vi "Scratch.vi"() -> ()   [LabVIEW 2020, in "VolatusGUIElements.lvlib" / "2WayValveV.lvclass"]
uses:
  2WayValveV.lvclass
  2WayValveV.lvclass/2WayValveV.ctl
  VolatusGUIControls/2WayValveH.ctl
  VolatusGUIControls/VolatusGUIControls.lvlib
  Picture.ctl
  Command Pictures.ctl
  Feedback Pictures.ctl
  Energized Pictures.ctl
  Valve Pictures.ctl
  Values.ctl
  Channel State.ctl
  Unused Element.ctl
panel:
  in  "Unused":T1
  in  "Valve Pictures":T2={"Command"={"Error"=enum."InError", "Config"=enum."InConfig", "Stale"=enum."InStale", "Close"=enum."InClose", "Open"=enum."InOpen", "TranClose"=enum."Blank", "TranOpen"=enum."Blank"}, "Feedback"={"Error"=enum."OutError", "Config"=enum."OutConfig", "Stale"=enum."OutStale", "Closed"=enum."OutClose", "Open"=enum."OutOpen", "TranClose"=enum."OutTranClose", "TranOpen"=enum."Blank"}, "Energized"={"Error"=enum."EnError", "Config"=enum."EnConfig", "Stale"=enum."EnStale", "False"=enum."EnOff", "True"=enum."EnOn"}}
  in  "Values":T7={"Command"={"Value"=FALSE, "Stale"=FALSE, "Config"=FALSE, "Error"=FALSE, "Prev"=FALSE}, "CmdFB"={"Value"=FALSE, "Stale"=FALSE, "Config"=FALSE, "Error"=FALSE, "Prev"=FALSE}, "Closed"={"Value"=TRUE, "Stale"=FALSE, "Config"=FALSE, "Error"=FALSE, "Prev"=FALSE}, "Open"={"Value"=FALSE, "Stale"=FALSE, "Config"=FALSE, "Error"=FALSE, "Prev"=FALSE}, "Energized"={"Value"=FALSE, "Stale"=FALSE, "Config"=FALSE, "Error"=FALSE, "Prev"=FALSE}}
  in  "2WayValve":T9={"Picture"=bytes[12402], "Command"=FALSE}
  # "Abort to stop"
  # "Config options below"
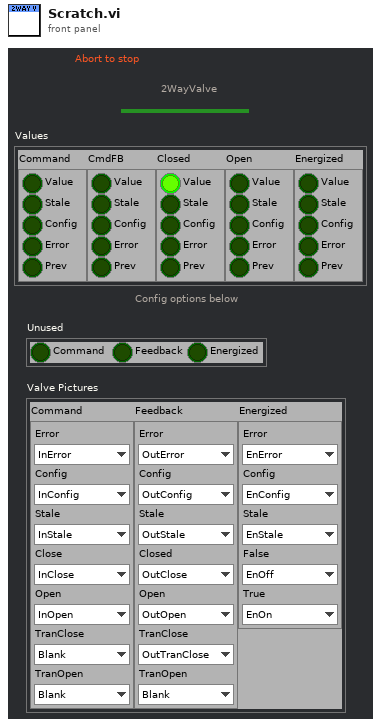
[diagram p1: front panel]
types:
  T1 = typedef "VolatusGUIElements.lvlib/2WayValveV.lvclass/Unused Element.ctl" = cluster{"Command":bool, "Feedback":bool, "Energized":bool}
  T2 = typedef "VolatusGUIElements.lvlib/2WayValveV.lvclass/Valve Pictures.ctl" = cluster{"Command":T3, "Feedback":T5, "Energized":T6}
  T3 = typedef "VolatusGUIElements.lvlib/2WayValveV.lvclass/Command Pictures.ctl" = cluster{"Error":T4, "Config":T4, "Stale":T4, "Close":T4, "Open":T4, "TranClose":T4, "TranOpen":T4}
  T4 = typedef "VolatusGUIElements.lvlib/2WayValveV.lvclass/Picture.ctl" = enum16{"Blank", "OutClose", "OutOpen", "OutTranClose", "OutTranOpen", "OutConfig", "OutStale", "OutError", "InClose", "InOpen", "InTranClose", "InTranOpen", "InConfig", "InStale", "InError", "EnOff", "EnOn", "EnConfig", "EnStale", "EnError"}
  T5 = typedef "VolatusGUIElements.lvlib/2WayValveV.lvclass/Feedback Pictures.ctl" = cluster{"Error":T4, "Config":T4, "Stale":T4, "Closed":T4, "Open":T4, "TranClose":T4, "TranOpen":T4}
  T6 = typedef "VolatusGUIElements.lvlib/2WayValveV.lvclass/Energized Pictures.ctl" = cluster{"Error":T4, "Config":T4, "Stale":T4, "False":T4, "True":T4}
  T7 = typedef "VolatusGUIElements.lvlib/2WayValveV.lvclass/Values.ctl" = cluster{"Command":T8, "CmdFB":T8, "Closed":T8, "Open":T8, "Energized":T8}
  T8 = typedef "VolatusGUIElements.lvlib/2WayValveV.lvclass/Channel State.ctl" = cluster{"Value":bool, "Stale":bool, "Config":bool, "Error":bool, "Prev":bool}
  T9 = typedef "VolatusGUIControls.lvlib/2WayValveH.ctl" = cluster{"Picture":picture, "Command":bool}
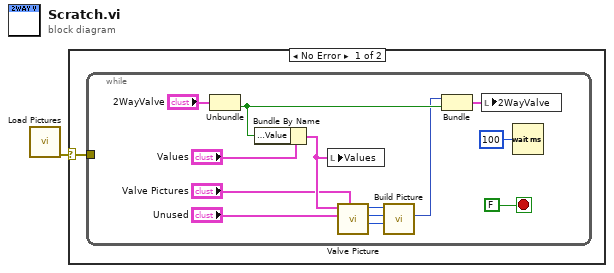
[diagram p0: block diagram]
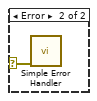
[diagram p2: hidden frame]
diagram:
  n1 = call "Load Pictures.vi"() -> ("error out"=w1:errorcluster)  [unwired: 11 in]
  n2 = case shown="No Error" w1 {
    selector: w1 -> [w2 w16]
    frame No Error {
      n3 = while {
        tunnel: w2 -> [_]
        stop <- FALSE stop-if-true
        n4 = Unbundle("2WayValve") -> ("Command"=w11:bool)  [unwired: 1 out]
        n5 = Bundle By Name(cluster="Values", "Command.Value"=w11) -> (w9:T7)
        n6 = local write "Values"(w9) -> ()
        n7 = call "Valve Picture.vi"("Valve Pictures"="Valve Pictures", "Unused Element"="Unused", "Values"=w9) -> ("Energized Picture"=w4:T4, "Feedback Picture"=w5:T4, "Command Picture"=w6:T4)  [unwired: 6 in]
        n8 = call "Build Picture.vi"("Energized Picture"=w4, "Feedback Picture"=w5, "Command Picture"=w6) -> ("Valve Picture"=w3:picture)  [unwired: 8 in]
        n9 = Bundle("Valve Picture"=w3, "Command"=w11) -> (w10:cluster{"Valve Picture":picture, "Command":bool})  [unwired: 1 in]
        n10 = local write "2WayValve"(w10) -> ()
        n11 = Wait (ms)(milliseconds to wait=u32 100) -> ()  [unwired: 1 out]
      }
    }
    frame Error {
      n12 = call <vilib>:"Simple Error Handler.vi"("error in (no error)"=w16) -> ()  [unwired: 4 in, 5 out]
    }
  }
